vi "Set Statut.vi"(8 "error in (no error)":errorcluster caption="entrée d'erreur (pas d'erreur)", 10 "Statut":enum16{"Erreur", "Close", "Open"}(ring), 11 "Class Shielding_ Box en entrée":refnum<class "Class Shielding_ Box (Default).lvclass">) -> (0 "error out":errorcluster caption="sortie d'erreur", 3 "Class Shielding_ Box en sortie":refnum<class "Class Shielding_ Box (Default).lvclass">)   [LabVIEW 2020, in "Library Instrument & Equipement.lvlib" / "Library Shielding box.lvlib" / "Class Shielding_ Box (Default).lvclass"]
uses:
  Class Shielding_ Box (Default).lvclass
  Class Shielding_ Box (Default).lvclass/Class Shielding_ Box (Default).ctl
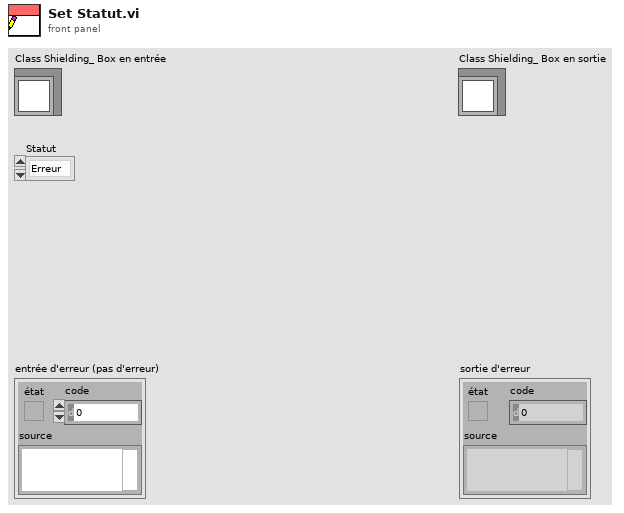
[diagram p1: front panel]
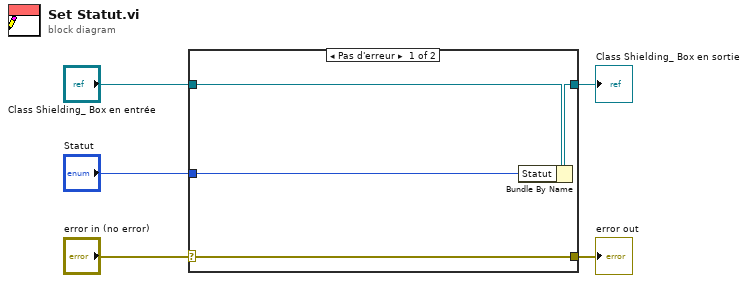
[diagram p0: block diagram]
diagram:
  n1 = case shown="Pas d'erreur" "error in (no error)" {
    selector: "error in (no error)" -> [w9 w10]
    tunnel: [w9 w10] -> w4
    tunnel: [w7 w11] -> w2
    tunnel: "Class Shielding_ Box en entrée" -> [w8 w11]
    tunnel: "Statut" -> [w6 _]
    frame No Error {
      n2 = Bundle By Name(cluster=w8, "Statut"=w6) -> (w7:refnum<class "Class Shielding_ Box (Default).lvclass">)
    }
    frame Error {
    }
  }
  "error out" <- w4
  "Class Shielding_ Box en sortie" <- w2
